vi "Core Action.vi"(8 "error in (no error)":errorcluster, 10 "SECS-II Class In":refnum<class "SECS-II Class.lvclass">, 11 "34-CEID Setup in":refnum<class "34-CEID Setup.lvclass">) -> (0 "error out":errorcluster, 2 "SECS-II Class Out":refnum<class "SECS-II Class.lvclass">, 3 "34-CEID Setup out":refnum<class "34-CEID Setup.lvclass">)   [LabVIEW 2020, in "SECS Scenarios.lvlib" / "34-CEID Setup.lvclass"]
uses:
  34-CEID Setup.lvclass
  D:/Dropbox/SECS/SECS_GEM v1.1.0/Com/SECS Scenarios/Scenarios Class/Scenarios Class.lvclass
  SECS Communication/SECS-II Class/SECS-II Class.lvclass
  SECS Communication/S2 Message Class/S2 Message Class.lvclass
  D:/Dropbox/SECS/SECS_GEM v1.1.0/Com/SECS Communication/SECS-II Class/SECS-II Class.lvclass
  Scenarios Class/Reply State.ctl
  Scenarios Class/Scenarios Class.lvclass/Scenarios Class.ctl
  Scenarios Class/Write Reply State.vi
  Scenarios Class/Read HSMS Class.vi
  SECS Communication/HSMS Class/HSMS Class.lvclass
  Scenarios Class/Scenarios Class.lvclass
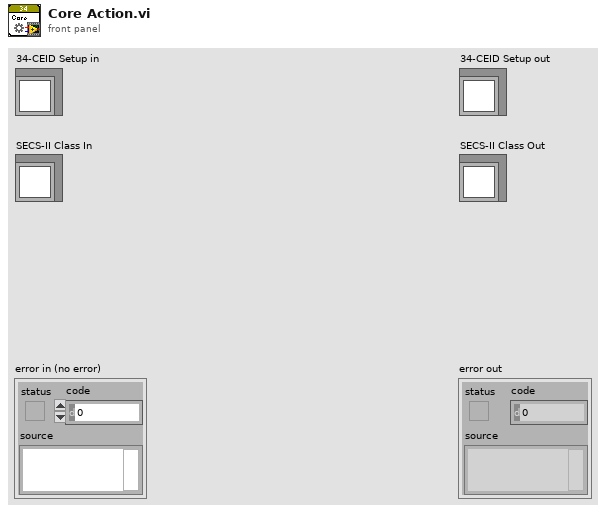
[diagram p1: front panel]
types:
  T1 = typedef "SECS Communication.lvlib/S2 Message Class.lvclass/S2F35.ctl" = cluster{"DATAID":u32, "CEID Data":cluster{"CEID":u32, "RPTID":u32[]}[]}
  T2 = typedef "SECS Scenarios.lvlib/Scenarios Class.lvclass/Reply State.ctl" = enum16{"OK", "Illegal Data", "Unknown Stream", "Unknown Function", "Off-Line", "T3 Timeout", "Inner-Timeout"}
  T3 = typedef "SECS Communication.lvlib/S2 Message Class.lvclass/S2F36.ctl" = enum16{"ok", "out of space", "invalid format", "1 or more CEID links already defined", "1 or more CEID invalid", "1 or more RPTID invalid"}
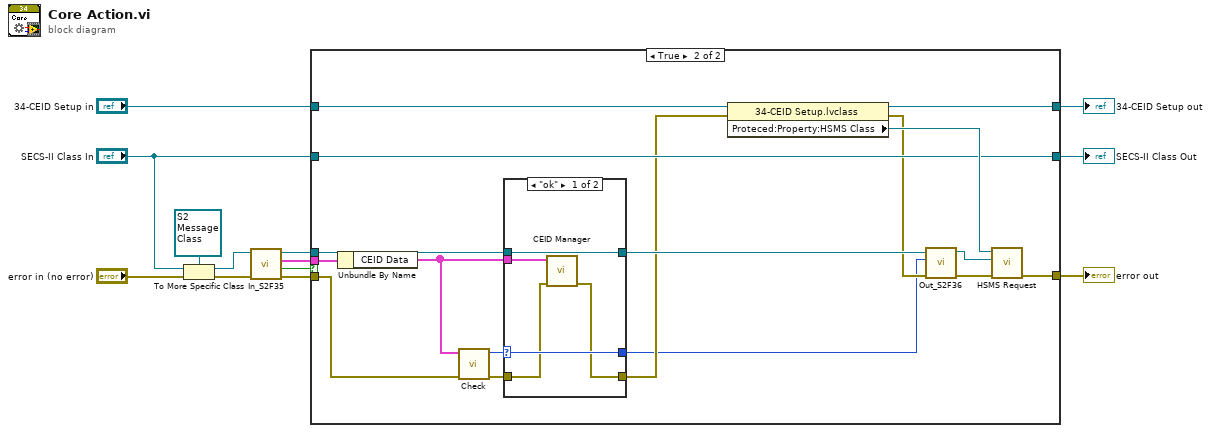
[diagram p0: block diagram]
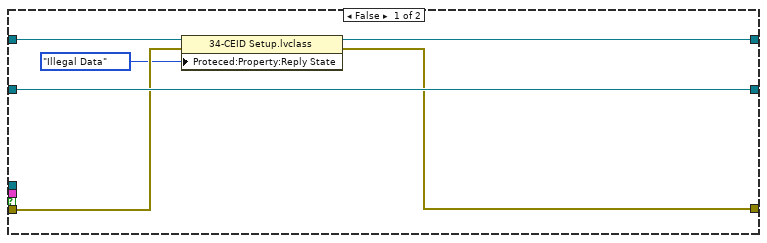
[diagram p2: hidden frame]
diagram:
  n1 = To More Specific Class(target class=refnum<class "S2 Message Class.lvclass"> refnum ("S2 Message Class in"), reference="SECS-II Class In", error in="error in (no error)") -> (specific class reference=w11:refnum<class "S2 Message Class.lvclass">, error out=w12:errorcluster)
  n2 = call "In_S2F35.vi"("error in (no error)"=w12, "S2 Message Class in"=w11) -> ("error out"=w9:errorcluster, "OK?"=w10:bool, "S2F35"=w8:T1, "S2 Message Class out"=w7:refnum<class "S2 Message Class.lvclass">)  [unwired: 6 in]
  n3 = case shown="True" w10 {
    tunnel: w9 -> [w17 w22]
    tunnel: w8 -> [_ w25]
    tunnel: w7 -> [_ w29]
    tunnel: "34-CEID Setup in" -> [w18 w36]
    tunnel: "SECS-II Class In" -> [w19 w33]
    tunnel: [w15 w34] -> w3
    tunnel: [w19 w33] -> w2
    tunnel: [w14 w32] -> w1
    frame False {
      n4 = property class="34-CEID Setup.lvclass"(reference=w18, error in=w17, "Proteced:Property:Reply State"=Reply_State."Illegal Data" ("Reply State")) -> (reference out=w15:refnum<class "34-CEID Setup.lvclass">, error out=w14:errorcluster)
    }
    frame True {
      n5 = Unbundle By Name(w25) -> ("CEID Data"=w23:cluster{"CEID":u32, "RPTID":u32[]}[])
      n6 = call "Check.vi"("error in (no error)"=w22, "CEID Data"=w23) -> ("error out"=w21:errorcluster, "S2F36"=w24:T3)  [unwired: 8 in]
      n7 = case shown="\"ok\"" w24 {
        selector: w24 -> [w40 w43]
        tunnel: w21 -> [w38 w44]
        tunnel: w29 -> [w41 w42]
        tunnel: [w37 w44] -> w27
        tunnel: [w40 w43] -> w20
        tunnel: [w41 w42] -> w28
        tunnel: w23 -> [w39 _]
        frame "ok" {
          n8 = call "CEID Manager.vi"("error in (no error)"=w38, "CEID Data"=w39) -> ("error out"=w37:errorcluster)  [unwired: 9 in]
        }
        frame Default {
        }
      }
      n9 = property class="34-CEID Setup.lvclass"(reference=w36, error in=w27) -> (reference out=w34:refnum<class "34-CEID Setup.lvclass">, error out=w26:errorcluster, "Proteced:Property:HSMS Class"=w35:refnum<class "HSMS Class.lvclass">)
      n10 = call "Out_S2F36.vi"("error in (no error)"=w26, "S2F36"=w20, "S2 Message Class in"=w28) -> ("error out"=w30:errorcluster, "S2 Message Class out"=w31:refnum<class "S2 Message Class.lvclass">)  [unwired: 7 in]
      n11 = call "HSMS Request.vi"("error in (no error)"=w30, "SECS-II Class In"=w31, "HSMS Class in"=w35) -> ("error out"=w32:errorcluster)  [unwired: 7 in, 1 out]
    }
  }
  "error out" <- w1
  "34-CEID Setup out" <- w3
  "SECS-II Class Out" <- w2
